vi "calibrate_offset_sliders.vi"(8 "error in (no error)":errorcluster, 10 "trajectory bounding box":refnum<class "Box.lvclass">, 11 "DL090202ScanHead in":refnum<class "ScanHeadDL090202.lvclass">) -> (0 "error out":errorcluster, 3 "DL090202ScanHead out":refnum<class "ScanHeadDL090202.lvclass">)   [LabVIEW 2010, in "ScanHeadDL090202.lvclass"]
uses:
  ScanHeadDL090202.lvclass
  common/classes/Box/Box/Box.lvclass
  ScanHeadDL090202.lvclass/ScanHeadDL090202.ctl
  common/classes/ErrorController/ErrorController/class_data.vi
  common/classes/SpaceVector/SpaceVector/SpaceVector.lvclass
  common/classes/ErrorController/ErrorController/ErrorController.lvclass
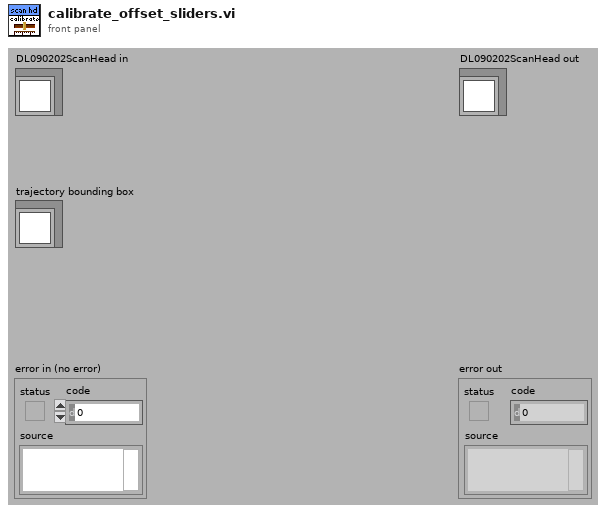
[diagram p1: front panel]
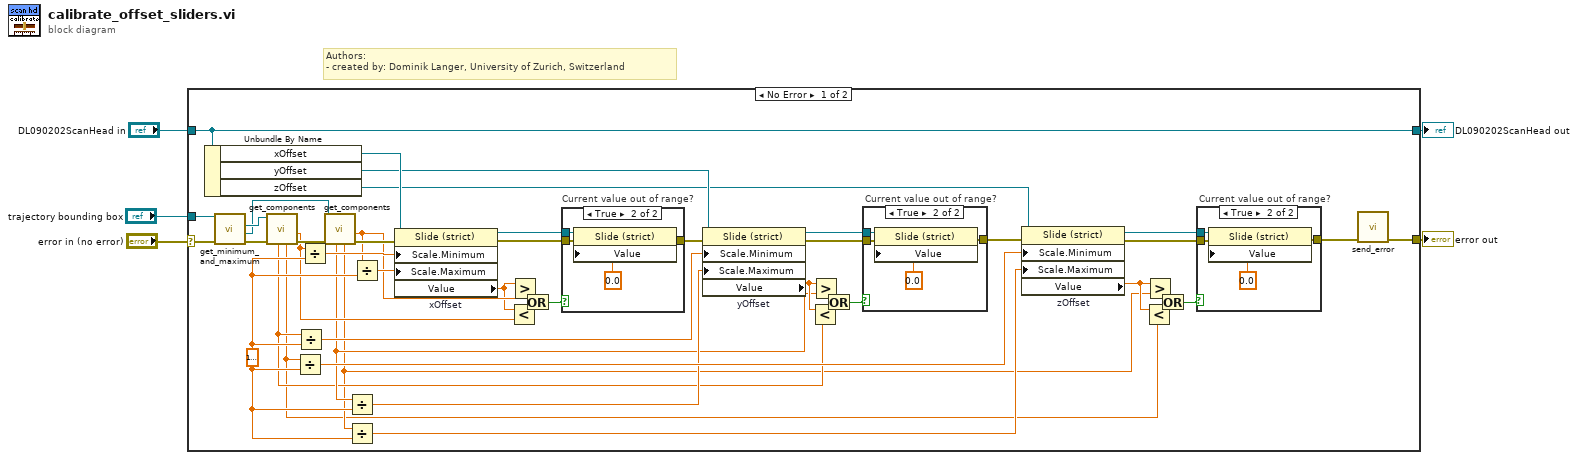
[diagram p0: block diagram]
diagram:
  # "Authors: \n- created by: Dominik Langer, University of Zurich, Switzerland"
  n1 = case shown="No Error" "error in (no error)" {
    selector: "error in (no error)" -> [w50 w68]
    tunnel: [w7 w68] -> w4
    tunnel: [w47 w67] -> w2
    tunnel: "DL090202ScanHead in" -> [w47 w67]
    tunnel: "trajectory bounding box" -> [w51 _]
    frame No Error {
      w37 = dbl[unit] 1e-06 ("Value")
      n2 = Unbundle By Name(w47) -> ("xOffset"=w44:refnum<vi>, "yOffset"=w42:refnum<vi>, "zOffset"=w41:refnum<vi>)
      n3 = call "get_minimum_and_maximum.vi"("error in (no error)"=w50, "Box in"=w51) -> ("error out"=w49:errorcluster, "maximum"=w45:refnum<class "SpaceVector.lvclass">, "minimum"=w46:refnum<class "SpaceVector.lvclass">)  [unwired: 7 out]
      n4 = call "get_components.vi"("error in (no error)"=w49, "SpaceVector in"=w46) -> ("error out"=w48:errorcluster, "x"=w31:dbl[unit], "z"=w8:dbl[unit], "y"=w16:dbl[unit])  [unwired: 6 out]
      n5 = Divide(x=w8, y=w37) -> (x/y=w38:dbl)
      n6 = Divide(x=w16, y=w37) -> (x/y=w39:dbl)
      n7 = Divide(x=w31, y=w37) -> (x/y=w40:dbl)
      n8 = call "get_components.vi"("error in (no error)"=w48, "SpaceVector in"=w45) -> ("error out"=w43:errorcluster, "x"=w33:dbl[unit], "z"=w9:dbl[unit], "y"=w17:dbl[unit])  [unwired: 6 out]
      n9 = Divide(x=w17, y=w37) -> (x/y=w36:dbl)
      n10 = Divide(x=w9, y=w37) -> (x/y=w35:dbl)
      n11 = Divide(x=w33, y=w37) -> (x/y=w34:dbl)
      n12 = property on="xOffset" class="Slide (strict)"(reference=w44, error in=w43, "Scale.Minimum"=w40, "Scale.Maximum"=w34) -> (reference out=w30:refnum<vi>, error out=w29:errorcluster, "Value"=w32:dbl[unit])
      n13 = Less?(x=w32, y=w31) -> (x < y?=w27:bool)
      n14 = Greater?(x=w32, y=w33) -> (0:w26:bool)
      n15 = Or(x=w26, y=w27) -> (x .or. y?=w25:bool)
      n16 = case "Current value out of range?" shown="True" w25 {
        tunnel: w30 -> [_ w66]
        tunnel: w29 -> [w62 w65]
        tunnel: [w62 w64] -> w28
        frame False {
        }
        frame True {
          n17 = property class="Slide (strict)"(reference=w66, error in=w65, "Value"=dbl[unit] 0.0) -> (error out=w64:errorcluster)  [unwired: 1 out]
        }
      }
      n18 = property on="yOffset" class="Slide (strict)"(reference=w42, error in=w28, "Scale.Minimum"=w39, "Scale.Maximum"=w36) -> (reference out=w20:refnum<vi>, error out=w21:errorcluster, "Value"=w19:dbl[unit])
      n19 = Less?(x=w19, y=w16) -> (x < y?=w24:bool)
      n20 = Greater?(x=w19, y=w17) -> (0:w23:bool)
      n21 = Or(x=w23, y=w24) -> (x .or. y?=w22:bool)
      n22 = case "Current value out of range?" shown="True" w22 {
        tunnel: w20 -> [_ w61]
        tunnel: w21 -> [w57 w60]
        tunnel: [w57 w59] -> w18
        frame False {
        }
        frame True {
          n23 = property class="Slide (strict)"(reference=w61, error in=w60, "Value"=dbl[unit] 0.0) -> (error out=w59:errorcluster)  [unwired: 1 out]
        }
      }
      n24 = property on="zOffset" class="Slide (strict)"(reference=w41, error in=w18, "Scale.Minimum"=w38, "Scale.Maximum"=w35) -> (reference out=w11:refnum<vi>, error out=w12:errorcluster, "Value"=w10:dbl[unit])
      n25 = Less?(x=w10, y=w8) -> (x < y?=w15:bool)
      n26 = Greater?(x=w10, y=w9) -> (0:w14:bool)
      n27 = Or(x=w14, y=w15) -> (x .or. y?=w13:bool)
      n28 = case "Current value out of range?" shown="True" w13 {
        tunnel: w11 -> [_ w56]
        tunnel: w12 -> [w52 w55]
        tunnel: [w52 w54] -> w6
        frame False {
        }
        frame True {
          n29 = property class="Slide (strict)"(reference=w56, error in=w55, "Value"=dbl[unit] 0.0) -> (error out=w54:errorcluster)  [unwired: 1 out]
        }
      }
      n30 = call "send_error.vi"("error in (no error)"=w6) -> ("error out"=w7:errorcluster)  [unwired: 10 in]
    }
    frame Error {
    }
  }
  "error out" <- w4
  "DL090202ScanHead out" <- w2
